vi "Main.vi"(7 "sweep rate, /min":dbl=0.2, 8 "sweep to:":dbl=4.0, 9 "sweep":T8(radio)=enum."2636a_smub") -> ()   [LabVIEW 2021] (continued)
            n5000 = property on="FieldRate(T/min)" class="DigNum (strict)"() -> ("Value"=w6385:dbl)  [unwired: 2 in, 2 out]
            n5001 = Divide(x=w6386, y=w6385) -> (x/y=w6384:dbl)
            n5002 = Multiply(x=w6384, y=60.0) -> (x*y=w6382:dbl)
          }
          frame "V2400_1_Step".."iTC_step", Default {
          }
        }
        n5003 = property on="Wait Between Step(s)" class="DigNum (strict)"() -> ("Value"=w6371:i32)  [unwired: 2 in, 2 out]
        n5004 = Add(x=w6375, y=w6374) -> (x+y=w6373:dbl)
        n5005 = Multiply(x=w6373, y=60.0) -> (x*y=w6372:dbl)
        n5006 = property on="HyperLoop Steps" class="Tbl (strict)"() -> ("Value"=w6352:string[][])  [unwired: 2 in, 2 out]
        n5007 = property on="wait between sweeps(s)" class="DigNum (strict)"() -> ("Value"=w6369:u32)  [unwired: 2 in, 2 out]
        n5008 = Add(x=w6372, y=w6371) -> (x+y=w6370:dbl)
        n5009 = property on="Step values" class="Tbl (strict)"() -> ("Value"=w6366:string[][])  [unwired: 2 in, 2 out]
        n5010 = Array Size(array=w6352) -> (size(s)=w6354:i32[])
        n5011 = Array Size(array=w6366) -> (size(s)=w6365:i32[])
        n5012 = Add(x=w6370, y=w6369) -> (x+y=w6359:dbl)
        n5013 = Index Array(array=w6354, index=0) -> (element=w6355:i32)
        n5014 = Index Array(array=w6365, index=0) -> (element=w6364:i32)
        n5015 = Add(x=w6359, y=w6356) -> (x+y=w6358:dbl)
        n5016 = Multiply(x=w6364, y=w6358) -> (x*y=w6351:dbl)
        n5017 = Multiply(x=w6355, y=w6351) -> (x*y=w6350:dbl)
        n5018 = Get Date/Time In Seconds() -> (seconds since 1Jan1904=w6368:timestamp)
        n5019 = Add(x=w6350, y=w6368) -> (x+y=w6346:timestamp)
        n5020 = Quotient & Remainder(x=w6350, y=3600.0) -> (x-y*floor(x/y)=w6367:dbl, floor(x/y)=w6347:dbl)
        n5021 = Quotient & Remainder(x=w6367, y=60.0) -> (x-y*floor(x/y)=w6349:dbl, floor(x/y)=w6348:dbl)
        n5022 = property on="Finish Time 2" class="AbsTime (strict)"("Value"=w6346) -> ()  [unwired: 2 in, 2 out]
        n5023 = property on="HH:" class="DigNum (strict)"("Value"=w6347) -> ()  [unwired: 2 in, 2 out]
        n5024 = property on="MM:" class="DigNum (strict)"("Value"=w6348) -> ()  [unwired: 2 in, 2 out]
        n5025 = property on="SS:" class="DigNum (strict)"("Value"=w6349) -> ()  [unwired: 2 in, 2 out]
      }
      event "EstimateTime": Value Change {
        n5026 = event-data() -> ()  [unwired: 1 in, 6 out]
        n5027 = property on="upper limit" class="DigNum (strict)"() -> ("Value"=w6417:dbl)  [unwired: 2 in, 2 out]
        n5028 = property on="lower limit" class="DigNum (strict)"() -> ("Value"=w6418:dbl)  [unwired: 2 in, 2 out]
        n5029 = Subtract(x=w6418, y=w6417) -> (x-y=w6416:dbl)
        n5030 = property on="Down Rate" class="DigNum (strict)"() -> ("Value"=w6413:dbl)  [unwired: 2 in, 2 out]
        n5031 = property on="Up Rate" class="DigNum (strict)"() -> ("Value"=w6415:dbl)  [unwired: 2 in, 2 out]
        n5032 = Absolute Value(x=w6416) -> (abs(x)=w6414:dbl)
        n5033 = property on="step" class="RadioBtnsControl (strict)"() -> ("Value"=w6392:T5)  [unwired: 2 in, 2 out]
        n5034 = Divide(x=w6414, y=w6415) -> (x/y=w6412:dbl)
        n5035 = Divide(x=w6414, y=w6413) -> (x/y=w6411:dbl)
        n5036 = case shown="\"iPS_step\"" w6392 {
          tunnel: [w6419 0.0] -> w6390
          frame "iPS_step" {
            n5037 = property on="step" class="DigNum (strict)"() -> ("Value"=w6423:dbl)  [unwired: 2 in, 2 out]
            n5038 = property on="FieldRate(T/min)" class="DigNum (strict)"() -> ("Value"=w6422:dbl)  [unwired: 2 in, 2 out]
            n5039 = Divide(x=w6423, y=w6422) -> (x/y=w6421:dbl)
            n5040 = Multiply(x=w6421, y=60.0) -> (x*y=w6419:dbl)
          }
          frame "V2400_1_Step".."iTC_step", Default {
          }
        }
        n5041 = property on="Wait Between Step(s)" class="DigNum (strict)"() -> ("Value"=w6408:i32)  [unwired: 2 in, 2 out]
        n5042 = Add(x=w6412, y=w6411) -> (x+y=w6410:dbl)
        n5043 = Multiply(x=w6410, y=60.0) -> (x*y=w6409:dbl)
        n5044 = property on="Step values" class="Tbl (strict)"() -> ("Value"=w6399:string[][])  [unwired: 2 in, 2 out]
        n5045 = property on="wait between sweeps(s)" class="DigNum (strict)"() -> ("Value"=w6406:u32)  [unwired: 2 in, 2 out]
        n5046 = Add(x=w6409, y=w6408) -> (x+y=w6407:dbl)
        n5047 = Array Size(array=w6399) -> (size(s)=w6398:i32[])
        n5048 = Index Array(array=w6398, index=0) -> (element=w6388:i32)
        n5049 = Add(x=w6407, y=w6406) -> (x+y=w6391:dbl)
        n5050 = Add(x=w6391, y=w6390) -> (x+y=w6389:dbl)
        n5051 = Get Date/Time In Seconds() -> (seconds since 1Jan1904=w6405:timestamp)
        n5052 = Multiply(x=w6388, y=w6389) -> (x*y=w6404:dbl)
        n5053 = Add(x=w6404, y=w6405) -> (x+y=w6396:timestamp)
        n5054 = Quotient & Remainder(x=w6404, y=3600.0) -> (x-y*floor(x/y)=w6403:dbl, floor(x/y)=w6395:dbl)
        n5055 = Quotient & Remainder(x=w6403, y=60.0) -> (x-y*floor(x/y)=w6393:dbl, floor(x/y)=w6394:dbl)
        n5056 = property on="SS:" class="DigNum (strict)"("Value"=w6393) -> ()  [unwired: 2 in, 2 out]
        n5057 = property on="MM:" class="DigNum (strict)"("Value"=w6394) -> ()  [unwired: 2 in, 2 out]
        n5058 = property on="HH:" class="DigNum (strict)"("Value"=w6395) -> ()  [unwired: 2 in, 2 out]
        n5059 = property on="Finish Time" class="AbsTime (strict)"("Value"=w6396) -> ()  [unwired: 2 in, 2 out]
      }
      event "Stop Mapping": Value Change {
        n5060 = event-data() -> ()  [unwired: 1 in, 6 out]
        n5061 = Flush Queue(queue=w6427) -> (queue out=w6428:refnum<queue>)  [unwired: 1 in, 2 out]
        n5062 = Enqueue Element(queue=w6428, element="Idle") -> ()  [unwired: 2 in, 3 out]
        n5063 = property on="Start Mapping" class="Bool"("DisabledEnum"=T10."Enabled" ("Disabled")) -> ()  [unwired: 2 in, 2 out]
        n5064 = property on="Stop Mapping" class="Bool"("DisabledEnum"=T10."Disabled and Grayed Out" ("Disabled")) -> ()  [unwired: 2 in, 2 out]
      }
      event "Stop HyperLoop": Value Change {
        n5065 = event-data() -> ()  [unwired: 1 in, 6 out]
        n5066 = Flush Queue(queue=w6432) -> (queue out=w6433:refnum<queue>)  [unwired: 1 in, 2 out]
        n5067 = Enqueue Element(queue=w6433, element="Idle") -> ()  [unwired: 2 in, 3 out]
        n5068 = property on="Start HyperLoop" class="Bool"("DisabledEnum"=T10."Enabled" ("Disabled")) -> ()  [unwired: 2 in, 2 out]
        n5069 = property on="Stop HyperLoop" class="Bool"("DisabledEnum"=T10."Disabled and Grayed Out" ("Disabled")) -> ()  [unwired: 2 in, 2 out]
      }
      event "Stop SuperHyper": Value Change {
        n5070 = event-data() -> ()  [unwired: 1 in, 6 out]
        n5071 = Flush Queue(queue=w6437) -> (queue out=w6438:refnum<queue>)  [unwired: 1 in, 2 out]
        n5072 = Enqueue Element(queue=w6438, element="Idle") -> ()  [unwired: 2 in, 3 out]
        n5073 = property on="StartSuperHyper" class="Bool"("DisabledEnum"=T10."Enabled" ("Disabled")) -> ()  [unwired: 2 in, 2 out]
        n5074 = property on="Stop SuperHyper" class="Bool"("DisabledEnum"=T10."Disabled and Grayed Out" ("Disabled")) -> ()  [unwired: 2 in, 2 out]
      }
      event "Sweep Down": Value Change {
        n5075 = event-data() -> ()  [unwired: 1 in, 6 out]
        n5076 = stacked-sequence {
          tunnel: w6440 -> [_ w6445]
          frame #0 {
            n5077 = property on="Down Rate" class="DigNum (strict)"() -> ("Value"=w6441:dbl)  [unwired: 2 in, 2 out]
            n5078 = property on="lower limit" class="DigNum (strict)"() -> ("Value"=w6442:dbl)  [unwired: 2 in, 2 out]
            n5079 = property on="sweep rate, /min" class="DigNum (strict)"("Value"=w6441) -> ()  [unwired: 2 in, 2 out]
            n5080 = property on="sweep to:" class="DigNum (strict)"("Value"=w6442) -> ()  [unwired: 2 in, 2 out]
            n5081 = property on="Sweep Down" class="Bool"("DisabledEnum"=T10."Disabled and Grayed Out" ("Disabled")) -> ()  [unwired: 2 in, 2 out]
          }
          frame #1 {
            n5082 = Flush Queue(queue=w6445) -> (queue out=w6444:refnum<queue>)  [unwired: 1 in, 2 out]
            n5083 = Enqueue Element(queue=w6444, element="Start Sweep") -> ()  [unwired: 2 in, 3 out]
          }
        }
      }
      event "Sweep Up": Value Change {
        n5084 = event-data() -> ()  [unwired: 1 in, 6 out]
        n5085 = stacked-sequence {
          tunnel: w6447 -> [_ w6452]
          frame #0 {
            w6448 = T10."Disabled and Grayed Out" ("Disabled")
            n5086 = property on="Up Rate" class="DigNum (strict)"() -> ("Value"=w6449:dbl)  [unwired: 2 in, 2 out]
            n5087 = property on="upper limit" class="DigNum (strict)"() -> ("Value"=w6450:dbl)  [unwired: 2 in, 2 out]
            n5088 = property on="sweep rate, /min" class="DigNum (strict)"("Value"=w6449) -> ()  [unwired: 2 in, 2 out]
            n5089 = property on="sweep to:" class="DigNum (strict)"("Value"=w6450) -> ()  [unwired: 2 in, 2 out]
            n5090 = property on="Sweep Down" class="Bool"("DisabledEnum"=w6448) -> ()  [unwired: 2 in, 2 out]
            n5091 = property on="Sweep Up" class="Bool"("DisabledEnum"=w6448) -> ()  [unwired: 2 in, 2 out]
          }
          frame #1 {
            n5092 = Flush Queue(queue=w6452) -> (queue out=w6451:refnum<queue>)  [unwired: 1 in, 2 out]
            n5093 = Enqueue Element(queue=w6451, element="Start Sweep") -> ()  [unwired: 2 in, 3 out]
          }
        }
      }
      event "Ramp\n Down": Value Change {
        n5094 = event-data() -> ()  [unwired: 1 in, 6 out]
        n5095 = Flush Queue(queue=w6455) -> (queue out=w6454:refnum<queue>)  [unwired: 1 in, 2 out]
        n5096 = property on="lower limit" class="DigNum (strict)"() -> ("Value"=w6458:dbl)  [unwired: 2 in, 2 out]
        n5097 = property on="Down Rate" class="DigNum (strict)"() -> ("Value"=w6457:dbl)  [unwired: 2 in, 2 out]
        n5098 = Enqueue Element(queue=w6454, element="Ramp To Limit") -> ()  [unwired: 2 in, 3 out]
        n5099 = property on="sweep to:" class="DigNum (strict)"("Value"=w6458) -> ()  [unwired: 2 in, 2 out]
        n5100 = property on="sweep rate, /min" class="DigNum (strict)"("Value"=w6457) -> ()  [unwired: 2 in, 2 out]
      }
      event "Ramp \nUp": Value Change {
        n5101 = event-data() -> ()  [unwired: 1 in, 6 out]
        n5102 = Flush Queue(queue=w6460) -> (queue out=w6459:refnum<queue>)  [unwired: 1 in, 2 out]
        n5103 = property on="Up Rate" class="DigNum (strict)"() -> ("Value"=w6461:dbl)  [unwired: 2 in, 2 out]
        n5104 = property on="upper limit" class="DigNum (strict)"() -> ("Value"=w6462:dbl)  [unwired: 2 in, 2 out]
        n5105 = Enqueue Element(queue=w6459, element="Ramp To Limit") -> ()  [unwired: 2 in, 3 out]
        n5106 = property on="sweep rate, /min" class="DigNum (strict)"("Value"=w6461) -> ()  [unwired: 2 in, 2 out]
        n5107 = property on="sweep to:" class="DigNum (strict)"("Value"=w6462) -> ()  [unwired: 2 in, 2 out]
      }
      event "Start Mapping", "HyperLoop Hidden": Value Change {
        n5108 = event-data() -> ()  [unwired: 1 in, 6 out]
        n5109 = stacked-sequence {
          tunnel: w6464 -> [_ _ _ _ w6551]
          frame #0 {
            n5110 = property on="Change Sweep Range" class="Bool (strict)"() -> ("Value"=w6465:bool)  [unwired: 2 in, 2 out]
            n5111 = case shown="True" w6465 {
              frame False {
              }
              frame True {
                n5112 = property on="Down          Up" class="Tbl (strict)"("Active Cell"=cluster{"Row":i32, "Column":i32} {"Row"=-2, "Column"=-2}, "Cell BG Color"=u32 16448250 ("Active Cell:Cell Background Color")) -> ()  [unwired: 2 in, 2 out]
              }
            }
            n5113 = property on="Step values" class="Tbl (strict)"("Active Cell"=cluster{"Row":i32, "Column":i32} {"Row"=-2, "Column"=-2}, "Cell BG Color"=u32 16448250 ("Active Cell:Cell Background Color")) -> ()  [unwired: 2 in, 2 out]
          }
          frame #1 {
            # "If change sweep range for different step value, set the sweep range"
            n5114 = property on="Change Sweep Range" class="Bool (strict)"() -> ("Value"=w6470:bool)  [unwired: 2 in, 2 out]
            n5115 = case shown="True" w6470 {
              frame False {
              }
              frame True {
                w6474 = 0 ("disabled index (col)")
                n5116 = property on="Down          Up" class="Tbl (strict)"() -> ("Value"=w6475:string[][])  [unwired: 2 in, 2 out]
                n5117 = Index Array(array=w6475, index (row)=w6474, index (col)=w6474) -> (element=w6476:string)
                n5118 = Index Array(array=w6475, index (row)=w6474, index (col)=1 ("disabled index (col)")) -> (element=w6472:string)
                n5119 = Fract/Exp String To Number(string=w6476) -> (number=w6477:dbl)  [unwired: 3 in, 1 out]
                n5120 = Fract/Exp String To Number(string=w6472) -> (number=w6471:dbl)  [unwired: 3 in, 1 out]
                n5121 = property on="lower limit" class="DigNum (strict)"("Value"=w6477) -> ()  [unwired: 2 in, 2 out]
                n5122 = property on="upper limit" class="DigNum (strict)"("Value"=w6471) -> ()  [unwired: 2 in, 2 out]
              }
            }
          }
          frame #2 {
            n5123 = property on="lower limit" class="DigNum (strict)" props=["Value"]() -> ()  [unwired: 2 in, 3 out]
            n5124 = property on="Stop Mapping" class="Bool"("DisabledEnum"=T10."Enabled" ("Disabled")) -> ()  [unwired: 2 in, 2 out]
            n5125 = property on="upper limit" class="DigNum (strict)"() -> ("Value"=w6478:dbl)  [unwired: 2 in, 2 out]
            n5126 = property on="Down Rate" class="DigNum (strict)"() -> ("Value"=w6481:dbl)  [unwired: 2 in, 2 out]
            n5127 = property on="sweep to:" class="DigNum (strict)"("Value"=w6478) -> ()  [unwired: 2 in, 2 out]
            n5128 = property on="sweep rate, /min" class="DigNum (strict)"("Value"=w6481) -> ()  [unwired: 2 in, 2 out]
            n5129 = property on="Sweep Direction" class="Str"("Value"="Ramp Down" ("String"), "Text.TextColor"=u32 0 ("Text.Text Colors:Text Color")) -> ()  [unwired: 2 in, 2 out]
            n5130 = property on="Start Mapping" class="Bool"("DisabledEnum"=T10."Disabled and Grayed Out" ("Disabled")) -> ()  [unwired: 2 in, 2 out]
            n5131 = property on="Table Index" class="DigNum (strict)"("Value"=0.0 ("Table Index")) -> ()  [unwired: 2 in, 2 out]
          }
          frame #3 {
            n5132 = property on="HyperLoop" class="Bool (strict)"() -> ("Value"=w6485:bool)  [unwired: 2 in, 2 out]
            n5133 = case shown="False" w6485 {
              frame False {
                # "Reserve two name strings for new mapping data file:\none for up\none for down"
                n5134 = property on="Data Folder" class="Path"() -> ("Value"=w6487:path)  [unwired: 2 in, 2 out]
                n5135 = property on="MappingName" class="Str"() -> ("Value"=w6486:string)  [unwired: 2 in, 2 out]
                n5136 = stacked-sequence {
                  tunnel: w6487 -> [w6493 w6524]
                  tunnel: w6486 -> [w6492 w6523]
                  frame #0 {
                    # "Up mapping"
                    n5137 = property on="HyperLoop" class="Bool (strict)"() -> ("Value"=w6489:bool)  [unwired: 2 in, 2 out]
                    n5138 = case shown="False" w6489 {
                      tunnel: ["_up" w6504] -> w6488
                      frame False {
                      }
                      frame True {
                        n5139 = property on="step_hyper" class="RadioBtnsControl (strict)"() -> ("Value"=w6505:T6)  [unwired: 2 in, 2 out]
                        n5140 = case shown="\"iTC_HyperLoop\"" w6505 {
                          tunnel: ["_V2400=" ("string") "_V2400=" ("string") "_Va=" ("string") "_Vb=" ("string") "_t=" ("string") "_T=" ("string") "_B" ("string")] -> w6500
                          tunnel: ["V" ("string") "V" ("string") "V" ("string") "V" ("string") _ "K" ("string") "T" ("string")] -> w6499
                          frame "2400_1_HyperLoop", Default {
                          }
                          frame "2400_2_HyperLoop" {
                          }
                          frame "2636_smua_HyperLoop" {
                          }
                          frame "2636_smub_HyperLoop" {
                          }
                          frame "time_HyperLoop" {
                          }
                          frame "iTC_HyperLoop" {
                          }
                          frame "iPS_HyperLoop" {
                          }
                        }
                        n5141 = property on="Current Hyper Value" class="DigNum (strict)"() -> ("Value"=w6502:dbl)  [unwired: 2 in, 2 out]
                        n5142 = Number To Exponential String(number=w6502) -> (E-format string=w6501:string)  [unwired: 3 in]
                        n5143 = Concatenate Strings("_up" ("string"), w6500, w6501, w6499) -> (w6504:string)
                      }
                    }
                    n5144 = Concatenate Strings(w6492, w6488) -> (w6490:string)
                    n5145 = call "AutoNamerDatExtraArtem.vi"("SweepType"=w6490, "Custom User Path"=w6493) -> ("String"=w6496:string, "Path"=w6497:path)  [unwired: 2 in]
                    n5146 = Path To String(path=w6497) -> (string=w6495:string)
                    n5147 = Concatenate Strings(w6495, "\\", w6496) -> (→"UpNameString":string)
                  }
                  frame #1 {
                    # "Down mapping"
                    n5148 = property on="HyperLoop" class="Bool (strict)"() -> ("Value"=w6520:bool)  [unwired: 2 in, 2 out]
                    n5149 = case shown="False" w6520 {
                      tunnel: ["_down" w6535] -> w6519
                      frame False {
                      }
                      frame True {
                        n5150 = property on="step_hyper" class="RadioBtnsControl (strict)"() -> ("Value"=w6536:T6)  [unwired: 2 in, 2 out]
                        n5151 = case shown="\"iPS_HyperLoop\"" w6536 {
                          tunnel: ["_V2400=" ("string") "_V2400=" ("string") "_Va=" ("string") "_Vb=" ("string") "_t=" ("string") "_T=" ("string") "_B" ("string")] -> w6531
                          tunnel: ["V" ("string") "V" ("string") "V" ("string") "V" ("string") _ "K" ("string") "T" ("string")] -> w6530
                          frame "2400_1_HyperLoop", Default {
                          }
                          frame "2400_2_HyperLoop" {
                          }
                          frame "2636_smua_HyperLoop" {
                          }
                          frame "2636_smub_HyperLoop" {
                          }
                          frame "time_HyperLoop" {
                          }
                          frame "iTC_HyperLoop" {
                          }
                          frame "iPS_HyperLoop" {
                          }
                        }
                        n5152 = property on="Current Hyper Value" class="DigNum (strict)"() -> ("Value"=w6533:dbl)  [unwired: 2 in, 2 out]
                        n5153 = Number To Exponential String(number=w6533) -> (E-format string=w6532:string)  [unwired: 3 in]
                        n5154 = Concatenate Strings("_down" ("string"), w6531, w6532, w6530) -> (w6535:string)
                      }
                    }
                    n5155 = Concatenate Strings(w6523, w6519) -> (w6521:string)
                    n5156 = call "AutoNamerDatExtraArtem.vi"("SweepType"=w6521, "Custom User Path"=w6524) -> ("String"=w6527:string, "Path"=w6528:path)  [unwired: 2 in]
                    n5157 = Path To String(path=w6528) -> (string=w6526:string)
                    n5158 = Concatenate Strings(w6526, "\\", w6527) -> (→"DownNameString":string)
                  }
                }
              }
              frame True {
              }
            }
          }
          frame #4 {
            n5159 = Flush Queue(queue=w6551) -> (queue out=w6550:refnum<queue>)  [unwired: 1 in, 2 out]
            n5160 = Enqueue Element(queue=w6550, element="Ramp To Limit") -> ()  [unwired: 2 in, 3 out]
          }
        }
      }
      event "Start HyperLoop", "Super Hidden": Value Change {
        n5161 = event-data() -> ()  [unwired: 1 in, 6 out]
        n5162 = stacked-sequence {
          tunnel: w6553 -> [_ _ _ w6605]
          frame #0 {
            n5163 = property on="HyperLoop Steps" class="Tbl (strict)"("Active Cell"=cluster{"Row":i32, "Column":i32} {"Row"=-2, "Column"=-2}, "Cell BG Color"=u32 16448250 ("Active Cell:Cell Background Color")) -> ()  [unwired: 2 in, 2 out]
          }
          frame #1 {
            n5164 = property on="Stop HyperLoop" class="Bool"("DisabledEnum"=T10."Enabled" ("Disabled")) -> ()  [unwired: 2 in, 2 out]
            n5165 = property on="Sweep Direction_Hyper" class="Str"("Value"="Ramp Down" ("String"), "Text.TextColor"=u32 0 ("Text.Text Colors:Text Color")) -> ()  [unwired: 2 in, 2 out]
            n5166 = property on="HyperLoop Index" class="DigNum (strict)"("Value"=0.0 ("Table Index")) -> ()  [unwired: 2 in, 2 out]
            n5167 = property on="Start HyperLoop" class="Bool"("DisabledEnum"=T10."Disabled and Grayed Out" ("Disabled")) -> ()  [unwired: 2 in, 2 out]
          }
          frame #2 {
            n5168 = property on="SuperHyper" class="Bool (strict)"() -> ("Value"=w6561:bool)  [unwired: 2 in, 2 out]
            n5169 = case shown="False" w6561 {
              frame False {
                # "Reserve two name strings for new hyperloop mapping data file:\none for up\none for down"
                n5170 = property on="Data Folder" class="Path"() -> ("Value"=w6563:path)  [unwired: 2 in, 2 out]
                n5171 = property on="MappingName" class="Str"() -> ("Value"=w6562:string)  [unwired: 2 in, 2 out]
                n5172 = stacked-sequence {
                  tunnel: w6563 -> [w6572 w6592]
                  tunnel: w6562 -> [w6571 w6591]
                  frame #0 {
                    # "Up mapping"
                    n5173 = property on="step_hyper" class="RadioBtnsControl (strict)"() -> ("Value"=w6568:T6)  [unwired: 2 in, 2 out]
                    n5174 = case shown="\"2636_smua_HyperLoop\"" w6568 {
                      tunnel: ["_V2400" ("string") "_V2400" ("string") "_Va" ("string") "_Vb" ("string") "_t" ("string") "_T" ("string") "_B" ("string")] -> w6567
                      frame "2400_1_HyperLoop", Default {
                        (unwired) "V" ("string")
                      }
                      frame "2400_2_HyperLoop" {
                        (unwired) "V" ("string")
                      }
                      frame "2636_smua_HyperLoop" {
                        (unwired) "V" ("string")
                      }
                      frame "2636_smub_HyperLoop" {
                        (unwired) "V" ("string")
                      }
                      frame "time_HyperLoop" {
                      }
                      frame "iTC_HyperLoop" {
                      }
                      frame "iPS_HyperLoop" {
                        (unwired) "T" ("string")
                      }
                    }
                    n5175 = Concatenate Strings("_HyperLoop" ("string"), w6567, "_up" ("string")) -> (w6569:string)
                    n5176 = Concatenate Strings(w6571, w6569) -> (w6570:string)
                    n5177 = call "AutoNamerDatExtraArtem.vi"("SweepType"=w6570, "Custom User Path"=w6572) -> ("String"=w6575:string, "Path"=w6576:path)  [unwired: 2 in]
                    n5178 = Path To String(path=w6576) -> (string=w6574:string)
                    n5179 = Concatenate Strings(w6574, "\\", w6575) -> (w6564:string)
                    n5180 = property on="UpNameString" class="Str"("Value"=w6564) -> ()  [unwired: 2 in, 2 out]
                  }
                  frame #1 {
                    # "Down mapping"
                    n5181 = property on="step_hyper" class="RadioBtnsControl (strict)"() -> ("Value"=w6588:T6)  [unwired: 2 in, 2 out]
                    n5182 = case shown="\"2400_2_HyperLoop\"" w6588 {
                      tunnel: ["_V2400" ("string") "_V2400" ("string") "_Va" ("string") "_Vb" ("string") "_t" ("string") "_T" ("string") "_B" ("string")] -> w6587
                      frame "2400_1_HyperLoop", Default {
                        (unwired) "V" ("string")
                      }
                      frame "2400_2_HyperLoop" {
                        (unwired) "V" ("string")
                      }
                      frame "2636_smua_HyperLoop" {
                        (unwired) "V" ("string")
                      }
                      frame "2636_smub_HyperLoop" {
                        (unwired) "V" ("string")
                      }
                      frame "time_HyperLoop" {
                      }
                      frame "iTC_HyperLoop" {
                        (unwired) "K" ("string")
                      }
                      frame "iPS_HyperLoop" {
                      }
                    }
                    n5183 = Concatenate Strings("_HyperLoop" ("string"), w6587, "_down" ("string")) -> (w6589:string)
                    n5184 = Concatenate Strings(w6591, w6589) -> (w6590:string)
                    n5185 = call "AutoNamerDatExtraArtem.vi"("SweepType"=w6590, "Custom User Path"=w6592) -> ("String"=w6595:string, "Path"=w6596:path)  [unwired: 2 in]
                    n5186 = Path To String(path=w6596) -> (string=w6594:string)
                    n5187 = Concatenate Strings(w6594, "\\", w6595) -> (w6584:string)
                    n5188 = property on="DownNameString" class="Str"("Value"=w6584) -> ()  [unwired: 2 in, 2 out]
                  }
                }
              }
              frame True {
              }
            }
          }
          frame #3 {
            n5189 = Flush Queue(queue=w6605) -> (queue out=w6604:refnum<queue>)  [unwired: 1 in, 2 out]
            n5190 = Enqueue Element(queue=w6604, element="Step to Next HyperLoop Value") -> ()  [unwired: 2 in, 3 out]
          }
        }
      }
      event "StartSuperHyper": Value Change {
        n5191 = event-data() -> ()  [unwired: 1 in, 6 out]
        n5192 = stacked-sequence {
          tunnel: w6607 -> [_ _ _ w6658]
          frame #0 {
            n5193 = property on="SuperHyper Steps" class="Tbl (strict)"("Active Cell"=cluster{"Row":i32, "Column":i32} {"Row"=-2, "Column"=-2}, "Cell BG Color"=u32 16448250 ("Active Cell:Cell Background Color")) -> ()  [unwired: 2 in, 2 out]
          }
          frame #1 {
            n5194 = property on="Stop SuperHyper" class="Bool"("DisabledEnum"=T10."Enabled" ("Disabled")) -> ()  [unwired: 2 in, 2 out]
            n5195 = property on="SuperHyper_Index" class="DigNum (strict)"("Value"=0.0 ("Table Index")) -> ()  [unwired: 2 in, 2 out]
            n5196 = property on="StartSuperHyper" class="Bool"("DisabledEnum"=T10."Disabled and Grayed Out" ("Disabled")) -> ()  [unwired: 2 in, 2 out]
            n5197 = property on="Sweep Direction3" class="Str"("Value"="Ramp Down" ("String"), "Text.TextColor"=u32 0 ("Text.Text Colors:Text Color")) -> ()  [unwired: 2 in, 2 out]
          }
          frame #2 {
            # "Reserve two name strings for new hyperloop mapping data file:\none for up\none for down"
            n5198 = property on="Data Folder" class="Path"() -> ("Value"=w6616:path)  [unwired: 2 in, 2 out]
            n5199 = property on="MappingName" class="Str"() -> ("Value"=w6615:string)  [unwired: 2 in, 2 out]
            n5200 = stacked-sequence {
              tunnel: w6616 -> [w6625 w6645]
              tunnel: w6615 -> [w6624 w6644]
              frame #0 {
                # "Up mapping"
                n5201 = property on="Step_SuperHyper" class="RadioBtnsControl (strict)"() -> ("Value"=w6617:T7)  [unwired: 2 in, 2 out]
                n5202 = case shown="\"2400_1_SuperHyper\", Default" w6617 {
                  tunnel: ["_V2400" ("string") "_V2400" ("string") "_Va" ("string") "_Vb" ("string") "_t" ("string") "_T" ("string") "_B" ("string")] -> w6621
                  frame "2400_1_SuperHyper", Default {
                    (unwired) "V" ("string")
                  }
                  frame "2400_2_SuperHyper" {
                    (unwired) "V" ("string")
                  }
                  frame "2636_smua_SuperHyper" {
                    (unwired) "V" ("string")
                  }
                  frame "2636_smub_SuperHyper" {
                    (unwired) "V" ("string")
                  }
                  frame "time_SuperHyper" {
                  }
                  frame "iTC_SuperHyper" {
                  }
                  frame "iPS_SuperHyper" {
                    (unwired) "T" ("string")
                  }
                }
                n5203 = Concatenate Strings("_SuperHyper" ("string"), w6621, "_up" ("string")) -> (w6622:string)
                n5204 = Concatenate Strings(w6624, w6622) -> (w6623:string)
                n5205 = call "AutoNamerDatExtraArtem.vi"("SweepType"=w6623, "Custom User Path"=w6625) -> ("String"=w6628:string, "Path"=w6629:path)  [unwired: 2 in]
                n5206 = Path To String(path=w6629) -> (string=w6627:string)
                n5207 = Concatenate Strings(w6627, "\\", w6628) -> (w6618:string)
                n5208 = property on="UpNameString" class="Str"("Value"=w6618) -> ()  [unwired: 2 in, 2 out]
              }
              frame #1 {
                # "Down mapping"
                n5209 = property on="Step_SuperHyper" class="RadioBtnsControl (strict)"() -> ("Value"=w6637:T7)  [unwired: 2 in, 2 out]
                n5210 = case shown="\"2400_2_SuperHyper\"" w6637 {
                  tunnel: ["_V2400" ("string") "_V2400" ("string") "_Va" ("string") "_Vb" ("string") "_t" ("string") "_T" ("string") "_B" ("string")] -> w6641
                  frame "2400_1_SuperHyper", Default {
                    (unwired) "V" ("string")
                  }
                  frame "2400_2_SuperHyper" {
                    (unwired) "V" ("string")
                  }
                  frame "2636_smua_SuperHyper" {
                    (unwired) "V" ("string")
                  }
                  frame "2636_smub_SuperHyper" {
                    (unwired) "V" ("string")
                  }
                  frame "time_SuperHyper" {
                  }
                  frame "iTC_SuperHyper" {
                    (unwired) "K" ("string")
                  }
                  frame "iPS_SuperHyper" {
                  }
                }
                n5211 = Concatenate Strings("_SuperHyper" ("string"), w6641, "_down" ("string")) -> (w6642:string)
                n5212 = Concatenate Strings(w6644, w6642) -> (w6643:string)
                n5213 = call "AutoNamerDatExtraArtem.vi"("SweepType"=w6643, "Custom User Path"=w6645) -> ("String"=w6648:string, "Path"=w6649:path)  [unwired: 2 in]
                n5214 = Path To String(path=w6649) -> (string=w6647:string)
                n5215 = Concatenate Strings(w6647, "\\", w6648) -> (w6638:string)
                n5216 = property on="DownNameString" class="Str"("Value"=w6638) -> ()  [unwired: 2 in, 2 out]
              }
            }
          }
          frame #3 {
            n5217 = Flush Queue(queue=w6658) -> (queue out=w6657:refnum<queue>)  [unwired: 1 in, 2 out]
            n5218 = Enqueue Element(queue=w6657, element="Step to Next SuperHyper Value") -> ()  [unwired: 2 in, 3 out]
          }
        }
      }
      event "Monitor": Value Change {
        n5219 = event-data() -> ()  [unwired: 1 in, 6 out]
        n5220 = case shown="True" "Monitor" {
          frame True {
            w6661 = TRUE ("Visible")
            n5221 = property on="Figure_axis" class="Arr (strict)"("Visible"=w6661) -> ()  [unwired: 2 in, 2 out]
            n5222 = property on="data" class="Arr (strict)"("Visible"=w6661) -> ()  [unwired: 2 in, 2 out]
            n5223 = property on="formula_variables" class="Arr (strict)"("Visible"=w6661) -> ()  [unwired: 2 in, 2 out]
          }
          frame False {
            w6662 = FALSE ("Visible")
            n5224 = property on="Figure_axis" class="Arr (strict)"("Visible"=w6662) -> ()  [unwired: 2 in, 2 out]
            n5225 = property on="formula_variables" class="Arr (strict)"("Visible"=w6662) -> ()  [unwired: 2 in, 2 out]
            n5226 = property on="data" class="Arr (strict)"("Visible"=w6662) -> ()  [unwired: 2 in, 2 out]
          }
        }
      }
      event "TempCtrl", "MagnetCtrl": Value Change {
        n5227 = event-data() -> ("CtlRef"=w6675:refnum<vi>)  [unwired: 1 in, 5 out]
        n5228 = property class="Bool"(reference=w6675) -> ("Label.Text"=w6674:string)  [unwired: 1 in, 2 out]
        n5229 = case shown="\"TempCtrl\", Default" w6674 {
          tunnel: w6665 -> [w6682 w6685]
          tunnel: [w6681 w6684] -> w6673
          tunnel: [w6680 w6683] -> w6669
          frame "TempCtrl", Default {
            n5230 = property on="iPS_addr_sweep" class="VISAName"() -> ("Value"=w6680:refnum<visa-resource-name>)  [unwired: 2 in, 2 out]
            n5231 = Unbundle(w6682) -> ("vi reference"=w6681:refnum<vi>)  [unwired: 1 out]
          }
          frame "MagnetCtrl" {
            n5232 = Unbundle(w6685) -> ("vi reference"=w6684:refnum<vi>)  [unwired: 1 out]
            n5233 = property on="iPS_addr_sweep" class="VISAName"() -> ("Value"=w6683:refnum<visa-resource-name>)  [unwired: 2 in, 2 out]
          }
        }
        n5234 = invoke class="VI" method="FP.Open"(reference=w6673, "Activate"=TRUE ("Activate?")) -> (reference out=w6671:refnum<vi>)  [unwired: 3 in, 4 out]
        n5235 = invoke class="VI" method="Ctrl Val.Set"(reference=w6671, "Control Name"="VISA resource name", "Value"=w6669) -> (reference out=w6668:refnum<vi>)  [unwired: 2 in, 4 out]
        n5236 = property class="VI"(reference=w6668) -> (reference out=w6666:refnum<vi>, "Exec.State"=w6667:T22)  [unwired: 1 in, 1 out]
        n5237 = case shown="\"Idle\"" w6667 {
          tunnel: w6666 -> [w6676 w6679]
          tunnel: [w6676 w6677] -> w6664
          frame "Bad", Default {
          }
          frame "Idle" {
            n5238 = invoke class="VI" method="Run VI"(reference=w6679, "Wait until done"=FALSE ("Wait Until Done")) -> (reference out=w6677:refnum<vi>)  [unwired: 3 in, 4 out]
          }
        }
        n5239 = property class="VI"(reference=w6664, "Front Panel.IsFrontmost"=TRUE ("Front Panel Window:Is Frontmost")) -> ()  [unwired: 1 in, 2 out]
      }
      event "Lockin_Setup", "Cytec_Switch": Value Change {
        n5240 = event-data() -> ("CtlRef"=w6692:refnum<vi>)  [unwired: 1 in, 5 out]
        n5241 = property class="Bool"(reference=w6692) -> ("Label.Text"=w6691:string)  [unwired: 1 in, 2 out]
        n5242 = case shown="\"Cytec_Switch\", Default" w6691 {
          tunnel: w6690 -> [w6697 w6699]
          tunnel: [w6696 w6698] -> w6689
          frame "Cytec_Switch", Default {
            n5243 = Unbundle(w6697) -> ("vi reference"=w6696:refnum<vi>)  [unwired: 1 out]
          }
          frame "Lockin_Setup" {
            n5244 = Unbundle(w6699) -> ("vi reference"=w6698:refnum<vi>)  [unwired: 1 out]
          }
        }
        n5245 = invoke class="VI" method="FP.Open"(reference=w6689, "Activate"=TRUE ("Activate?")) -> (reference out=w6687:refnum<vi>)  [unwired: 3 in, 4 out]
        n5246 = property class="VI"(reference=w6687) -> (reference out=w6686:refnum<vi>, "Exec.State"=w6688:T22)  [unwired: 1 in, 1 out]
        n5247 = case shown="\"Idle\"" w6688 {
          tunnel: w6686 -> [_ w6694]
          frame "Bad", Default {
          }
          frame "Idle" {
            n5248 = invoke class="VI" method="Run VI"(reference=w6694, "Wait until done"=FALSE ("Wait Until Done")) -> ()  [unwired: 3 in, 5 out]
          }
        }
      }
    }
  }
  n5249 = Release Queue(queue=w4) -> ()  [unwired: 2 in, 3 out]
